vi "题目3.vi"() -> ()   [LabVIEW 2017]
panel:
  in  "停止":bool
  out "温度":string
  out "温度计":dbl(slide) scale=0.0..260.0
  in  "温度单位":bool
  # "℉"
  # "℃"
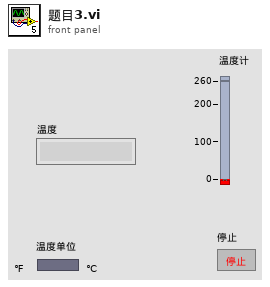
[diagram p1: front panel]
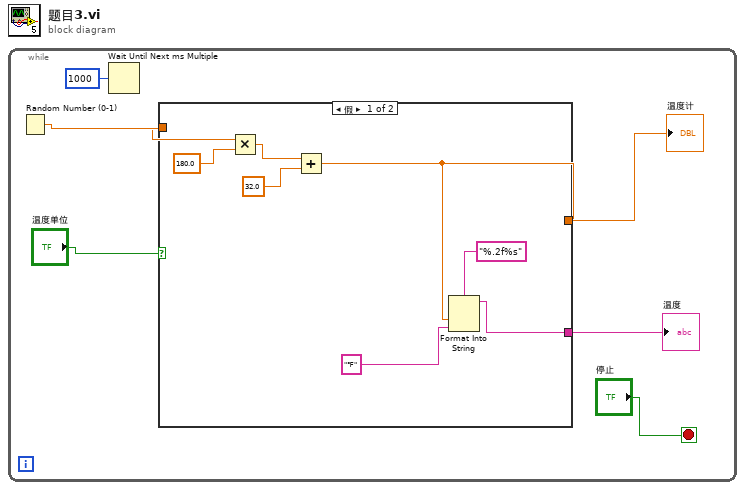
[diagram p0: block diagram]
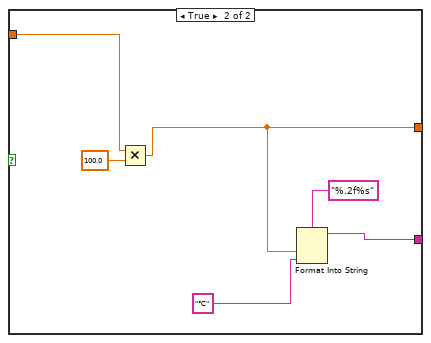
[diagram p2: hidden frame]
diagram:
  n1 = while {
    stop <- "停止" stop-if-true
    n2 = Random Number (0-1)() -> (number: 0 to 1=w2:dbl)
    n3 = Wait Until Next ms Multiple(millisecond multiple=u32 1000 ("毫秒倍数")) -> ()  [unwired: 1 out]
    n4 = case shown="假" "温度单位" {
      tunnel: [w8 w18] -> w6
      tunnel: [w7 w17] -> w5
      tunnel: w2 -> [w14 w15]
      frame False {
        n5 = Multiply(x=w14, y=180.0) -> (x*y=w12:dbl)
        n6 = Add(x=w12, y=32.0) -> (x+y=w8:dbl)
        n7 = Format Into String(format string="%.2f%s" ("格式字符串"), w8, "℉") -> (resulting string=w7:string)  [unwired: 2 in, 1 out]
      }
      frame True {
        n8 = Multiply(x=w15, y=100.0) -> (x*y=w18:dbl)
        n9 = Format Into String(format string="%.2f%s" ("格式字符串"), w18, "℃") -> (resulting string=w17:string)  [unwired: 2 in, 1 out]
      }
    }
    "温度计" <- w6
    "温度" <- w5
  }
